vi "SingleGraphCreation_DataCollection_WAVEFORM.vi"(9 "wfm":i16[][](array[numeric]), 10 "index":i32, 11 "wfm info":T1(array[cluster])) -> (2 "output waveform":waveform(dbl), 3 "Array":dbl[](array[numeric]))   [LabVIEW 2019]
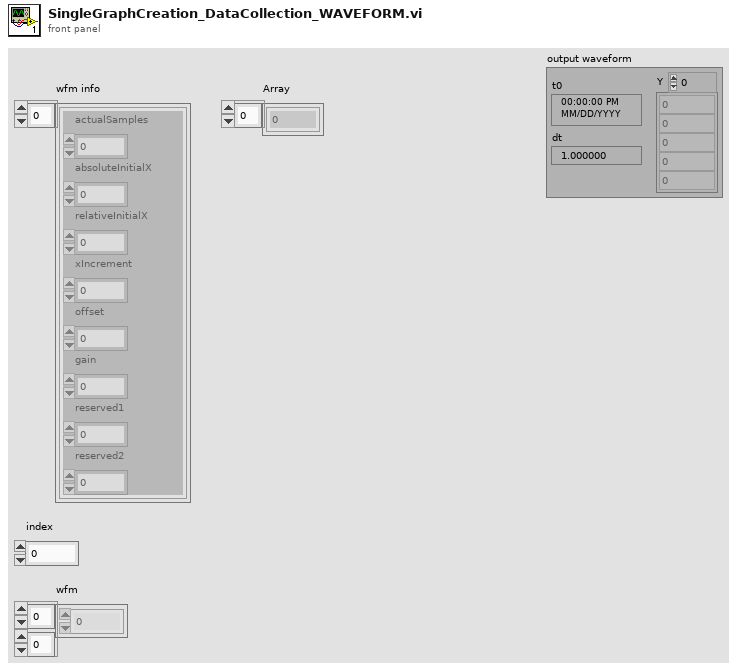
[diagram p1: front panel]
types:
  T1 = cluster{"actualSamples":i32, "absoluteInitialX":dbl, "relativeInitialX":dbl, "xIncrement":dbl, "offset":dbl, "gain":dbl, "reserved1":dbl, "reserved2":dbl}[]
  T2 = cluster{"actualSamples":i32, "absoluteInitialX":dbl, "relativeInitialX":dbl, "xIncrement":dbl, "offset":dbl, "gain":dbl, "reserved1":dbl, "reserved2":dbl}
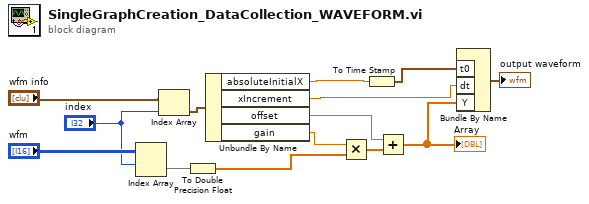
[diagram p0: block diagram]
diagram:
  n1 = Index Array(array="wfm", index (row)="index") -> (element=w10:i16[])  [unwired: 1 in]
  n2 = Index Array(array="wfm info", index="index") -> (element=w9:T2)
  n3 = To Double Precision Float(number=w10) -> (double precision float=w14:dbl[])
  n4 = Unbundle By Name(w9) -> ("absoluteInitialX"=w4:dbl, "xIncrement"=w1:dbl, "offset"=w12:dbl, "gain"=w13:dbl)
  n5 = Multiply(x=w13, y=w14) -> (x*y=w11:dbl[])
  n6 = To Time Stamp(1:w4) -> (0:w3:timestamp)
  n7 = Add(x=w12, y=w11) -> (x+y=w5:dbl[])
  "Array" <- w5
  n8 = Bundle By Name("t0"=w3, "dt"=w1, "Y"=w5) -> (→"output waveform":waveform(dbl))  [unwired: 1 in]
